vi "write_master_hbt.vi"(10 "hbt":u16, 11 "node":u8) -> (3 "return":i16)   [LabVIEW 2011]
uses:
  canopen_dll_master.dll
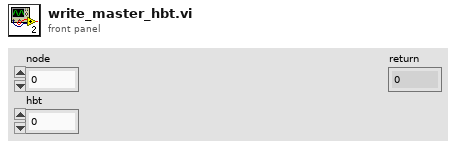
[diagram p1: front panel]
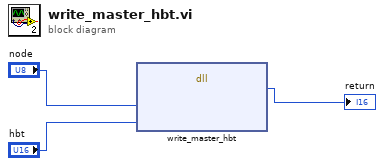
[diagram p0: block diagram]
diagram:
  n1 = dll-call lib="canopen_dll_master.dll" fn="write_master_hbt"("node"="node", "hbt"="hbt") -> ("return type"=→"return":i16)  [unwired: 5 in, 2 out]
